vi "LEDC Control Loop 2936 Init.vi"(0 "LEDAD Port":refnum<visa-resource-name>="COM7", 1 "Wavelength":string="1550", 5 "Light Meter Port":refnum<visa-resource-name>="COM4", 9 "Illumination Cal Factor":dbl=3.62982 format="%#.6f", 11 "error in (no error)":errorcluster, 12 "Unit":u16(ring) items=["nW/cm^2", "pW/cm^2"], 13 "Channel":enum16{"Chn1", "Chn2"}(ring)) -> (3 "In Progress":bool, 4 "LEDAD Port out":refnum<visa-resource-name>, 6 "Light Meter Port out":refnum<visa-resource-name>, 8 "WL>800":bool, 10 "Max Illum":dbl format="%#_4g", 14 "Done":bool, 15 "error out":errorcluster)   [LabVIEW 2010]
panel:
  # "nm"
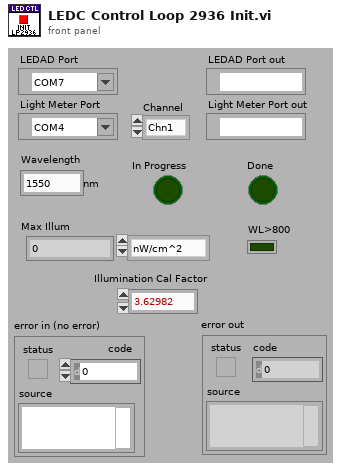
[diagram p1: front panel]
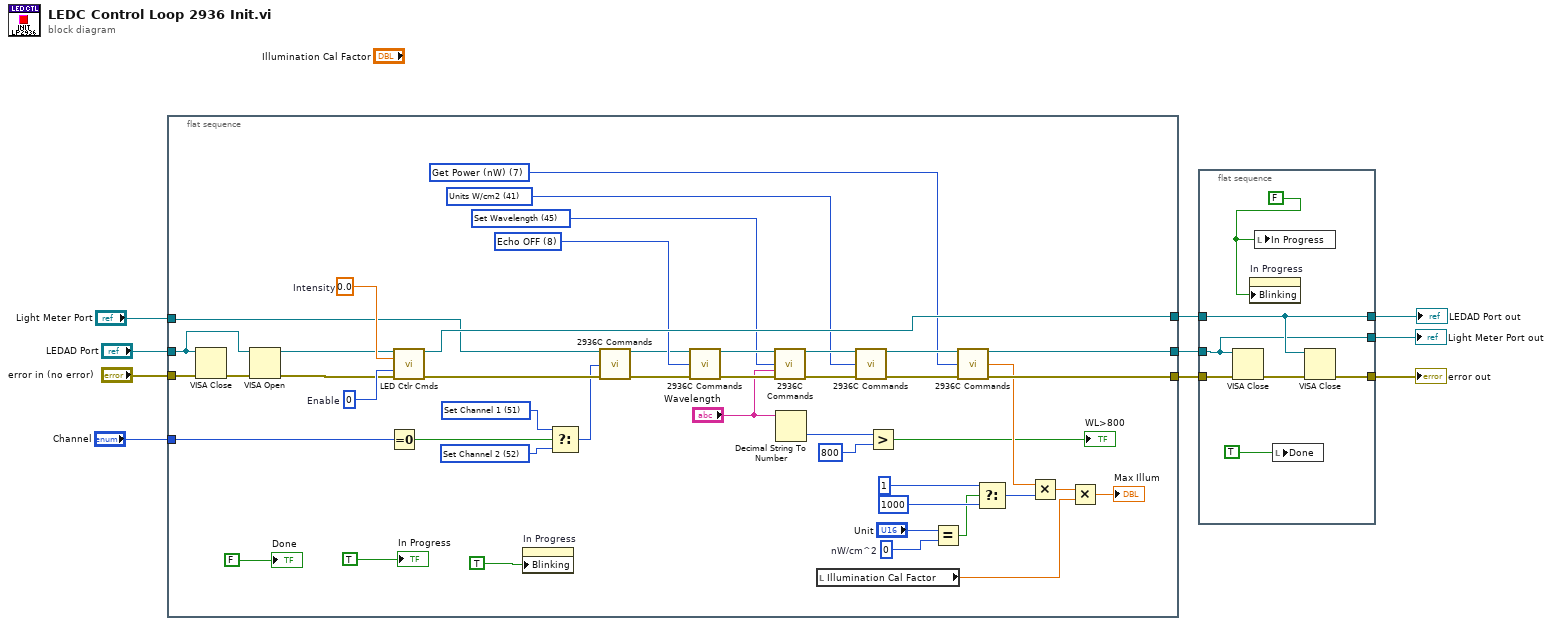
[diagram p0: block diagram]
diagram:
  n1 = flat-sequence {
    tunnel: "error in (no error)" -> [w56]
    tunnel: "LEDAD Port" -> [w54]
    tunnel: "Light Meter Port" -> [w18]
    tunnel: [w51] -> w3
    tunnel: [w50] -> w4
    tunnel: [w24] -> w2
    tunnel: "Channel" -> [w12]
    frame #0 {
      w14 = u16 52 items=["Attenuator OFF", "Attenuator ON", "Attenuator Query", "Beep OFF", "Beep ON", "Beep Query", "Clear Status Reg", "Get Power (nW)", "Echo OFF", "Echo ON", "Echo Query", "No Filter", "Analog Filter", "Digital FIlter", "Filter Query", "Hold", "Go", "Go Query", "Backlight OFF", "Backlight Medium", "Backlight High", "Backlight Query", "Set Dsplay Screen 0", "Set Display Screen 1", "Display Screen Query", "Mode DC Continuous", "Mode DC Single", "Mode Integrate", "Identification", "Auto Range", "Auto Range Query", "Signal Range 0", "Signal Range 1", "Signal Range 2", "Signal Range 3", "Signal Range 4", "Signal Range 5", "Signal Range 6", "Signal Range Query", "Store Reference", "Units W", "Units W/cm2", "Units dBm", "Units Joules", "Units Query", "Set Wavelength", "Wavelength Querry", "Mode Pesk-to-Peak Cont.", "Mode Peak-to-Peak Sing.", "Mode Query", "Channel Querry", "Set Channel 1", "Set Channel 2"] ("Command")
      w15 = u16 51 items=["Attenuator OFF", "Attenuator ON", "Attenuator Query", "Beep OFF", "Beep ON", "Beep Query", "Clear Status Reg", "Get Power (nW)", "Echo OFF", "Echo ON", "Echo Query", "No Filter", "Analog Filter", "Digital FIlter", "Filter Query", "Hold", "Go", "Go Query", "Backlight OFF", "Backlight Medium", "Backlight High", "Backlight Query", "Set Dsplay Screen 0", "Set Display Screen 1", "Display Screen Query", "Mode DC Continuous", "Mode DC Single", "Mode Integrate", "Identification", "Auto Range", "Auto Range Query", "Signal Range 0", "Signal Range 1", "Signal Range 2", "Signal Range 3", "Signal Range 4", "Signal Range 5", "Signal Range 6", "Signal Range Query", "Store Reference", "Units W", "Units W/cm2", "Units dBm", "Units Joules", "Units Query", "Set Wavelength", "Wavelength Querry", "Mode Pesk-to-Peak Cont.", "Mode Peak-to-Peak Sing.", "Mode Query", "Channel Querry", "Set Channel 1", "Set Channel 2"] ("Command")
      w20 = u16 7 items=["Attenuator OFF", "Attenuator ON", "Attenuator Query", "Beep OFF", "Beep ON", "Beep Query", "Clear Status Reg", "Get Power (nW)", "Echo OFF", "Echo ON", "Echo Query", "No Filter", "Analog Filter", "Digital FIlter", "Filter Query", "Hold", "Go", "Go Query", "Backlight OFF", "Backlight Medium", "Backlight High", "Backlight Query", "Set Dsplay Screen 0", "Set Display Screen 1", "Display Screen Query", "Mode DC Continuous", "Mode DC Single", "Mode Integrate", "Identification", "Auto Range", "Auto Range Query", "Signal Range 0", "Signal Range 1", "Signal Range 2", "Signal Range 3", "Signal Range 4", "Signal Range 5", "Signal Range 6", "Signal Range Query", "Store Reference", "Units W", "Units W/cm2", "Units dBm", "Units Joules", "Units Query", "Set Wavelength", "Wavelength Querry", "Mode Pesk-to-Peak Cont.", "Mode Peak-to-Peak Sing.", "Mode Query", "Channel Querry", "Set Channel 1", "Set Channel 2"] ("Command")
      w21 = u16 41 items=["Attenuator OFF", "Attenuator ON", "Attenuator Query", "Beep OFF", "Beep ON", "Beep Query", "Clear Status Reg", "Get Power (nW)", "Echo OFF", "Echo ON", "Echo Query", "No Filter", "Analog Filter", "Digital FIlter", "Filter Query", "Hold", "Go", "Go Query", "Backlight OFF", "Backlight Medium", "Backlight High", "Backlight Query", "Set Dsplay Screen 0", "Set Display Screen 1", "Display Screen Query", "Mode DC Continuous", "Mode DC Single", "Mode Integrate", "Identification", "Auto Range", "Auto Range Query", "Signal Range 0", "Signal Range 1", "Signal Range 2", "Signal Range 3", "Signal Range 4", "Signal Range 5", "Signal Range 6", "Signal Range Query", "Store Reference", "Units W", "Units W/cm2", "Units dBm", "Units Joules", "Units Query", "Set Wavelength", "Wavelength Querry", "Mode Pesk-to-Peak Cont.", "Mode Peak-to-Peak Sing.", "Mode Query", "Channel Querry", "Set Channel 1", "Set Channel 2"] ("Command")
      w22 = u16 45 items=["Attenuator OFF", "Attenuator ON", "Attenuator Query", "Beep OFF", "Beep ON", "Beep Query", "Clear Status Reg", "Get Power (nW)", "Echo OFF", "Echo ON", "Echo Query", "No Filter", "Analog Filter", "Digital FIlter", "Filter Query", "Hold", "Go", "Go Query", "Backlight OFF", "Backlight Medium", "Backlight High", "Backlight Query", "Set Dsplay Screen 0", "Set Display Screen 1", "Display Screen Query", "Mode DC Continuous", "Mode DC Single", "Mode Integrate", "Identification", "Auto Range", "Auto Range Query", "Signal Range 0", "Signal Range 1", "Signal Range 2", "Signal Range 3", "Signal Range 4", "Signal Range 5", "Signal Range 6", "Signal Range Query", "Store Reference", "Units W", "Units W/cm2", "Units dBm", "Units Joules", "Units Query", "Set Wavelength", "Wavelength Querry", "Mode Pesk-to-Peak Cont.", "Mode Peak-to-Peak Sing.", "Mode Query", "Channel Querry", "Set Channel 1", "Set Channel 2"] ("Command")
      w23 = u16 8 items=["Attenuator OFF", "Attenuator ON", "Attenuator Query", "Beep OFF", "Beep ON", "Beep Query", "Clear Status Reg", "Get Power (nW)", "Echo OFF", "Echo ON", "Echo Query", "No Filter", "Analog Filter", "Digital FIlter", "Filter Query", "Hold", "Go", "Go Query", "Backlight OFF", "Backlight Medium", "Backlight High", "Backlight Query", "Set Dsplay Screen 0", "Set Display Screen 1", "Display Screen Query", "Mode DC Continuous", "Mode DC Single", "Mode Integrate", "Identification", "Auto Range", "Auto Range Query", "Signal Range 0", "Signal Range 1", "Signal Range 2", "Signal Range 3", "Signal Range 4", "Signal Range 5", "Signal Range 6", "Signal Range Query", "Store Reference", "Units W", "Units W/cm2", "Units dBm", "Units Joules", "Units Query", "Set Wavelength", "Wavelength Querry", "Mode Pesk-to-Peak Cont.", "Mode Peak-to-Peak Sing.", "Mode Query", "Channel Querry", "Set Channel 1", "Set Channel 2"] ("Command")
      w44 = 0  # nW/cm^2
      w27 = u8 0  # Enable
      w28 = 0.0  # Intensity
      n2 = VISA Close(VISA resource name=w54, error in (no error)=w56) -> (error out=w55:errorcluster)
      n3 = VISA Open(error in (no error)=w55, VISA resource name=w54) -> (VISA resource name=w26:refnum<visa-resource-name>, error out=w25:errorcluster)  [unwired: 3 in]
      n4 = Equal To 0?(x=w12) -> (x = 0?=w11:bool)
      n5 = call "LED Ctlr Cmds.vi"("VISA session"=w26, "Intensity"=w28, "Enable"=w27, "error in (no error)"=w25) -> ("VISA session out"=w24:refnum<visa-resource-name>, "error out"=w19:errorcluster)  [unwired: 7 in, 3 out]
      n6 = property on="In Progress" class="Bool (strict)"("Blinking"=TRUE) -> ()  [unwired: 2 in, 2 out]
      n7 = Select(t=w15, s=w11, f=w14) -> (s? t:f=w13:u16)
      n8 = call "2936C Commands.vi"("Instrument Resource Name"=w18, "Command"=w13, "error in (no error)"=w19) -> ("VISA resource name out"=w17:refnum<visa-resource-name>, "error out"=w16:errorcluster)  [unwired: 8 in, 3 out]
      n9 = call "2936C Commands.vi"("Instrument Resource Name"=w17, "Command"=w23, "error in (no error)"=w16) -> ("VISA resource name out"=w52:refnum<visa-resource-name>, "error out"=w53:errorcluster)  [unwired: 8 in, 3 out]
      n10 = call "2936C Commands.vi"("Instrument Resource Name"=w52, "Command"=w22, "Wavelength"="Wavelength", "error in (no error)"=w53) -> ("VISA resource name out"=w39:refnum<visa-resource-name>, "error out"=w40:errorcluster)  [unwired: 7 in, 3 out]
      n11 = Decimal String To Number(string="Wavelength") -> (number=w36:i32)  [unwired: 2 in, 1 out]
      n12 = local read "Illumination Cal Factor"() -> (w30:dbl)
      n13 = call "2936C Commands.vi"("Instrument Resource Name"=w39, "Command"=w21, "error in (no error)"=w40) -> ("VISA resource name out"=w34:refnum<visa-resource-name>, "error out"=w32:errorcluster)  [unwired: 8 in, 3 out]
      n14 = Greater?(x=w36, y=800) -> (0:→"WL>800":bool)
      n15 = Equal?(x="Unit", y=w44) -> (x = y?=w43:bool)
      n16 = call "2936C Commands.vi"("Instrument Resource Name"=w34, "Command"=w20, "error in (no error)"=w32) -> ("VISA resource name out"=w51:refnum<visa-resource-name>, "LM Response"=w42:dbl, "error out"=w50:errorcluster)  [unwired: 8 in, 2 out]
      n17 = Select(t=1, s=w43, f=1000) -> (s? t:f=w38:i32)
      n18 = Multiply(x=w42, y=w38) -> (x*y=w31:dbl)
      n19 = Multiply(x=w31, y=w30) -> (x*y=→"Max Illum":dbl)
      "Done" <- FALSE
      "In Progress" <- TRUE
    }
  }
  n20 = flat-sequence {
    tunnel: w3 -> [w59]
    tunnel: w4 -> [w61]
    tunnel: [w60] -> w5
    tunnel: w2 -> [w60]
    tunnel: [w59] -> w6
    tunnel: [w57] -> w7
    frame #0 {
      w63 = FALSE
      n21 = VISA Close(VISA resource name=w59, error in (no error)=w61) -> (error out=w58:errorcluster)
      n22 = property on="In Progress" class="Bool (strict)"("Blinking"=w63) -> ()  [unwired: 2 in, 2 out]
      n23 = local write "In Progress"(w63) -> ()
      n24 = local write "Done"(TRUE) -> ()
      n25 = VISA Close(VISA resource name=w60, error in (no error)=w58) -> (error out=w57:errorcluster)
    }
  }
  "LEDAD Port out" <- w5
  "Light Meter Port out" <- w6
  "error out" <- w7
